vi "Set Infinite Timeouts.vi"(10 "infinite timeouts":bool, 11 "FIFO Debug Flags in":refnum<class "FIFO Flags.lvclass">) -> (3 "FIFO Debug Flags out":refnum<class "FIFO Flags.lvclass">)   [LabVIEW 2017, in "DSF Core.lvlib" / "FIFO Flags.lvclass"]
uses:
  FIFO Flags.lvclass
  FIFO Flags.lvclass/FIFO Flags.ctl
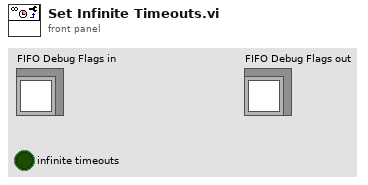
[diagram p1: front panel]
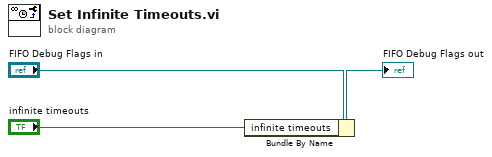
[diagram p0: block diagram]
diagram:
  n1 = Bundle By Name(cluster="FIFO Debug Flags in", "infinite timeouts"="infinite timeouts") -> (→"FIFO Debug Flags out":refnum<class "FIFO Flags.lvclass">)
